vi "UserID.vi"(8 "Error In":errorcluster, 11 "Path In":path) -> (0 "Error Out":errorcluster, 1 "Student Info":T1, 3 "Path Out":path)   [LabVIEW 2014]
uses:
  Ctls/Student Info.ctl
  <vilib>/regexp/Match Regular Expression.xnode
panel:
  out "Subject Number":bool=TRUE
  out "Student Full Name":bool=TRUE
  out "Student Class Number":bool=TRUE
  out "Student ID":bool=TRUE
  out "Warning Text":string
  in  "Subject Number":string caption="Disciplina"
  in  "Student Class Number":string caption="Turma"
  in  "Student Full Name":string caption="Nome Completo"
  in  "Student ID":string caption="Número USP"
  in  "OK":bool
  # "Dados do Usuário"
  # "Verifique / Preencha os campos abaixo referentes aos dados do usuário:"
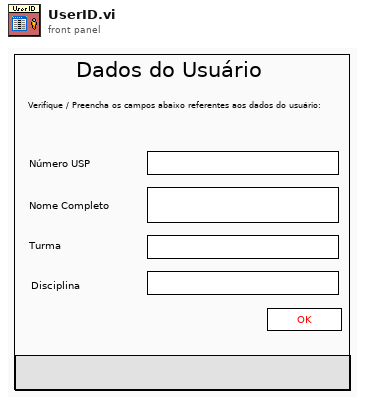
[diagram p1: front panel]
types:
  T1 = typedef "Student Info.ctl" = cluster{"Student ID":string, "Student Full Name":string, "Student Class Number":string, "Subject Number":string, "Last Online":string}
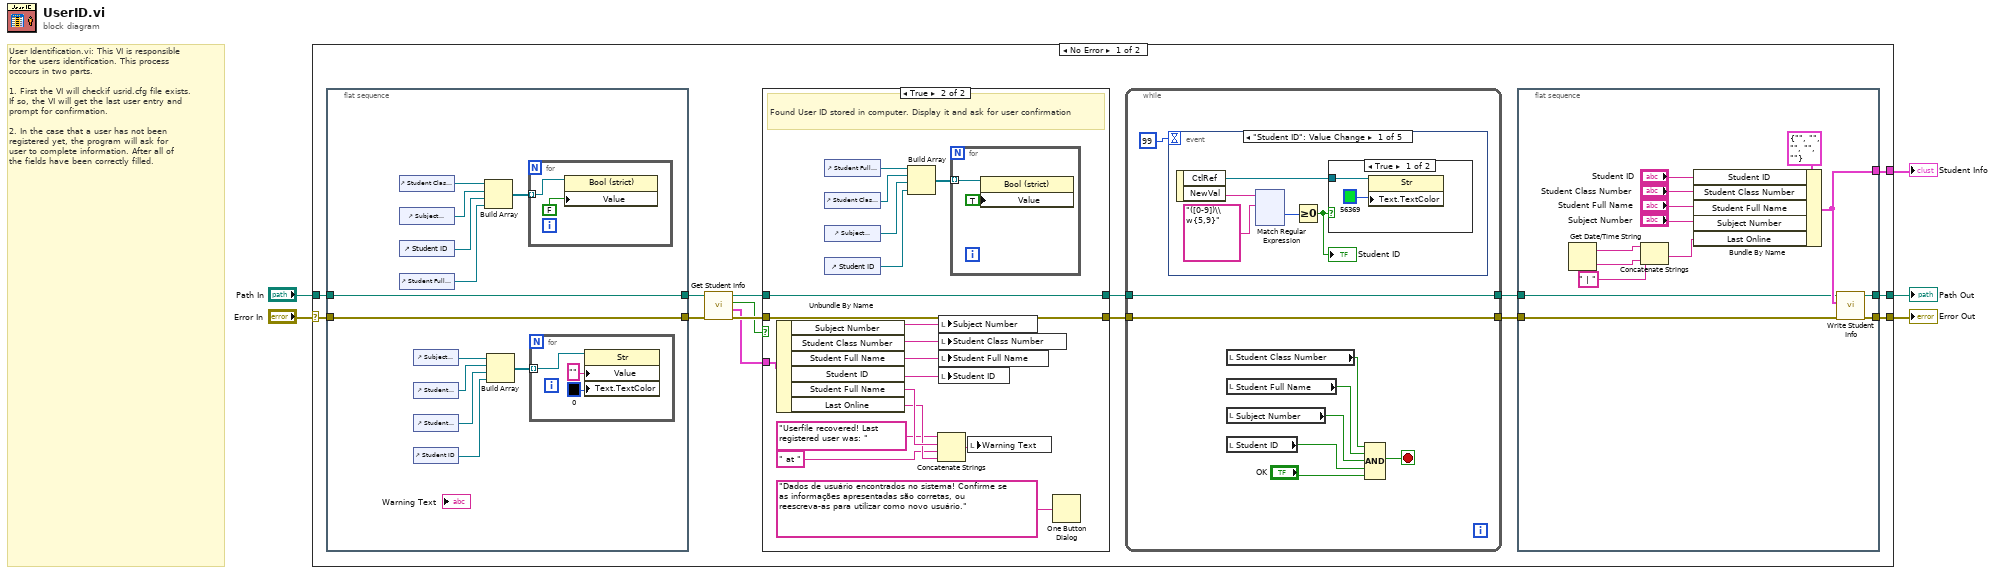
[diagram p0: block diagram]
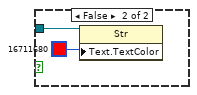
[diagram p2: hidden frame]
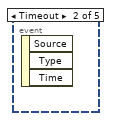
[diagram p3: hidden frame]
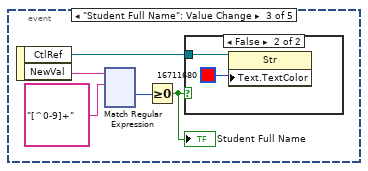
[diagram p4: hidden frame]
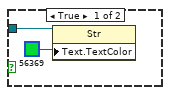
[diagram p5: hidden frame]
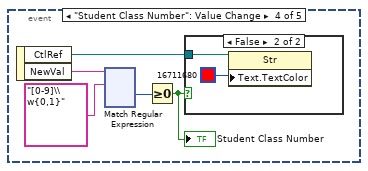
[diagram p6: hidden frame]
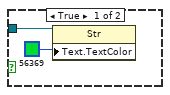
[diagram p7: hidden frame]
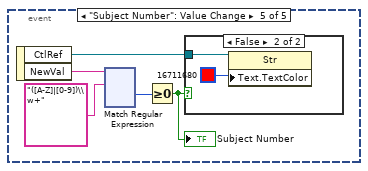
[diagram p8: hidden frame]
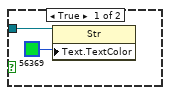
[diagram p9: hidden frame]
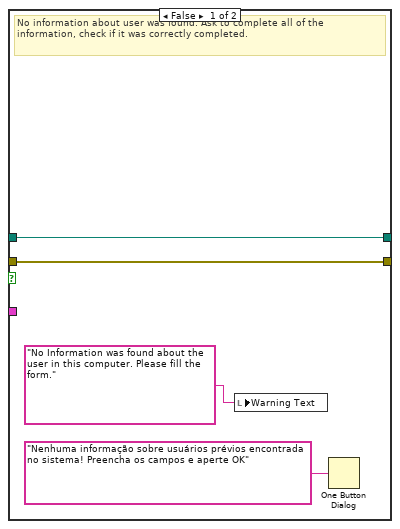
[diagram p10: hidden frame]
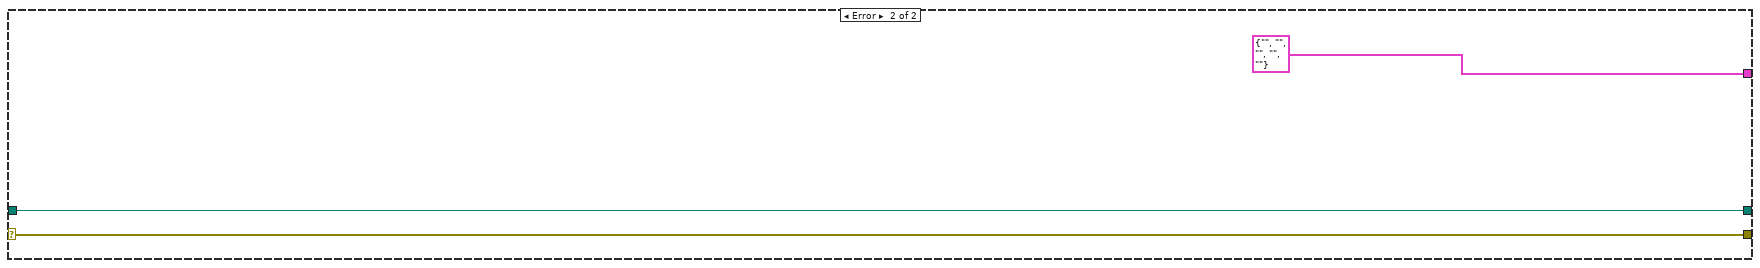
[diagram p11: hidden frame]
diagram:
  # "User Identification.vi: This VI is responsible \nfor the users identification. This process \noccours in two parts. \n\n1. First the VI will checkif usrid.cfg file exists.\nIf so, the VI will get the last user entry and \nprompt for confirmation.\n\n2. In the case that a user has not been \nregistered yet, the program will ask for\nuser to complete information. After all of \nthe fields have been correctly filled."
  n1 = case shown="No Error" "Error In" {
    selector: "Error In" -> [w15 w579]
    tunnel: [w11 w579] -> w5
    tunnel: "Path In" -> [w16 w578]
    tunnel: [w12 w578] -> w2
    tunnel: [w10 T1 {"Student ID"="", "Student Full Name"="", "Student Class Number"="", "Subject Number"="", "Last Online"=""} ("Student Info")] -> w1
    frame No Error {
      n2 = flat-sequence {
        tunnel: w16 -> [w537]
        tunnel: w15 -> [w536]
        tunnel: [w537] -> w14
        tunnel: [w536] -> w13
        frame #0 {
          n3 = control-ref of="Student Class Number"() -> (w541:refnum<vi>)
          n4 = control-ref of="Subject Number"() -> (w540:refnum<vi>)
          n5 = control-ref of="Student ID"() -> (w539:refnum<vi>)
          n6 = control-ref of="Student Full Name"() -> (w538:refnum<vi>)
          n7 = control-ref of="Subject Number"() -> (w545:refnum<vi>)
          n8 = control-ref of="Student Class Number"() -> (w544:refnum<vi>)
          n9 = control-ref of="Student Full Name"() -> (w543:refnum<vi>)
          n10 = control-ref of="Student ID"() -> (w542:refnum<vi>)
          n11 = Build Array(w541, w540, w539, w538) -> (w547:refnum<vi>[])
          n12 = Build Array(w545, w544, w543, w542) -> (w546:refnum<vi>[])
          n13 = for {
            tunnel: w547 -> [w549] mode=indexing
            n14 = property class="Bool (strict)"(reference=w549, "Value"=FALSE) -> ()  [unwired: 1 in, 2 out]
          }
          n15 = for {
            tunnel: w546 -> [w552] mode=indexing
            n16 = property class="Str"(reference=w552, "Value"="", "Text.TextColor"=u32 0) -> ()  [unwired: 1 in, 2 out]
          }
        }
      }
      n17 = call "Get Student Info.vi"("Error In"=w13, "Path In"=w14) -> ("Error Out"=w20:errorcluster, "Student Info"=w18:T1, "Found Usr Cfg File?"=w17:bool, "Path Out"=w19:path)  [unwired: 6 in]
      n18 = case shown="True" w17 {
        tunnel: [w555 w564] -> w9
        tunnel: w20 -> [w555 w564]
        tunnel: w19 -> [w556 w563]
        tunnel: w18 -> [_ w574]
        tunnel: [w556 w563] -> w8
        frame False {
          # "No information about user was found. Ask to complete all of the information, check if it was correctly completed."
          n19 = local write "Warning Text"("No Information was found about the user in this computer. Please fill the form." ("Warning Text")) -> ()
          n20 = One Button Dialog(message="Nenhuma informação sobre usuários prévios encontrada no sistema! Preencha os campos e aperte OK" ("regular expression")) -> ()  [unwired: 1 in, 1 out]
        }
        frame True {
          # "Found User ID stored in computer. Display it and ask for user confirmation"
          n21 = Unbundle By Name(w574) -> ("Subject Number"=w573:string, "Student Class Number"=w572:string, "Student Full Name"=w571:string, "Student ID"=w570:string, "Student Full Name"=w569:string, "Last Online"=w568:string)
          n22 = control-ref of="Student Full Name"() -> (w559:refnum<vi>)
          n23 = control-ref of="Student Class Number"() -> (w560:refnum<vi>)
          n24 = control-ref of="Subject Number"() -> (w561:refnum<vi>)
          n25 = control-ref of="Student ID"() -> (w562:refnum<vi>)
          n26 = Build Array(w559, w560, w561, w562) -> (w558:refnum<vi>[])
          n27 = Concatenate Strings("Userfile recovered! Last registered user was: ", w569, " at " ("string"), w568) -> (w565:string)
          n28 = local write "Subject Number"(w573) -> ()
          n29 = local write "Student Class Number"(w572) -> ()
          n30 = local write "Student Full Name"(w571) -> ()
          n31 = local write "Student ID"(w570) -> ()
          n32 = for {
            tunnel: w558 -> [w576] mode=indexing
            n33 = property class="Bool (strict)"(reference=w576, "Value"=TRUE) -> ()  [unwired: 1 in, 2 out]
          }
          n34 = local write "Warning Text"(w565) -> ()
          n35 = One Button Dialog(message="Dados de usuário encontrados no sistema! Confirme se as informações apresentadas são corretas, ou reescreva-as para utilizar como novo usuário." ("regular expression")) -> ()  [unwired: 1 in, 1 out]
        }
      }
      n36 = while {
        tunnel: w9 -> [w43]
        tunnel: [w43] -> w6
        tunnel: w8 -> [w40]
        tunnel: [w40] -> w7
        stop <- w41 stop-if-true
        n37 = event shown="[0] \"Student ID\": Value Change" {
          selector: _ -> [_ _ _ _ _]
          dyn-events: _ -> [_ _ _ _ _]
          timeout: 99 -> [_ _ _ _ _]
          event "Student ID": Value Change {
            n38 = event-data() -> ("CtlRef"=w48:refnum<vi>, "NewVal"=w44:string)  [unwired: 1 in]
            n39 = xnode "Match Regular Expression"("input string"=w44, "regular expression"="([0-9])\\w{5,9}") -> ("offset past match"=w45:i32)  [unwired: 4 in, 4 out]
            n40 = Greater Or Equal To 0?(x=w45) -> (x >= 0?=w46:bool)
            "Student ID" <- w46
            n41 = case shown="True" w46 {
              tunnel: w48 -> [w164 w165]
              frame True {
                n42 = property on="Property Node" class="Str"(reference=w164, "Text.TextColor"=u32 56369) -> ()  [unwired: 1 in, 2 out]
              }
              frame False {
                n43 = property on="Property Node" class="Str"(reference=w165, "Text.TextColor"=u32 16711680) -> ()  [unwired: 1 in, 2 out]
              }
            }
          }
          event Timeout {
            n44 = event-data() -> ()  [unwired: 1 in, 3 out]
          }
          event "Student Full Name": Value Change {
            n45 = event-data() -> ("CtlRef"=w168:refnum<vi>, "NewVal"=w169:string)  [unwired: 1 in]
            n46 = xnode "Match Regular Expression"("input string"=w169, "regular expression"="[^0-9]+") -> ("offset past match"=w170:i32)  [unwired: 4 in, 4 out]
            n47 = Greater Or Equal To 0?(x=w170) -> (x >= 0?=w167:bool)
            "Student Full Name" <- w167
            n48 = case shown="False" w167 {
              tunnel: w168 -> [w173 w174]
              frame True {
                n49 = property on="Property Node" class="Str"(reference=w173, "Text.TextColor"=u32 56369) -> ()  [unwired: 1 in, 2 out]
              }
              frame False {
                n50 = property on="Property Node" class="Str"(reference=w174, "Text.TextColor"=u32 16711680) -> ()  [unwired: 1 in, 2 out]
              }
            }
          }
          event "Student Class Number": Value Change {
            n51 = event-data() -> ("CtlRef"=w291:refnum<vi>, "NewVal"=w293:string)  [unwired: 1 in]
            n52 = xnode "Match Regular Expression"("input string"=w293, "regular expression"="[0-9]\\w{0,1}") -> ("offset past match"=w292:i32)  [unwired: 4 in, 4 out]
            n53 = Greater Or Equal To 0?(x=w292) -> (x >= 0?=w290:bool)
            "Student Class Number" <- w290
            n54 = case shown="False" w290 {
              tunnel: w291 -> [w296 w297]
              frame True {
                n55 = property on="Property Node" class="Str"(reference=w296, "Text.TextColor"=u32 56369) -> ()  [unwired: 1 in, 2 out]
              }
              frame False {
                n56 = property on="Property Node" class="Str"(reference=w297, "Text.TextColor"=u32 16711680) -> ()  [unwired: 1 in, 2 out]
              }
            }
          }
          event "Subject Number": Value Change {
            n57 = event-data() -> ("CtlRef"=w414:refnum<vi>, "NewVal"=w416:string)  [unwired: 1 in]
            n58 = xnode "Match Regular Expression"("input string"=w416, "regular expression"="([A-Z]|[0-9])\\w+") -> ("offset past match"=w415:i32)  [unwired: 4 in, 4 out]
            n59 = Greater Or Equal To 0?(x=w415) -> (x >= 0?=w413:bool)
            "Subject Number" <- w413
            n60 = case shown="False" w413 {
              tunnel: w414 -> [w419 w420]
              frame True {
                n61 = property on="Property Node" class="Str"(reference=w419, "Text.TextColor"=u32 56369) -> ()  [unwired: 1 in, 2 out]
              }
              frame False {
                n62 = property on="Property Node" class="Str"(reference=w420, "Text.TextColor"=u32 16711680) -> ()  [unwired: 1 in, 2 out]
              }
            }
          }
        }
        n63 = local read "Student Class Number"() -> (w36:bool)
        n64 = local read "Student Full Name"() -> (w37:bool)
        n65 = local read "Subject Number"() -> (w38:bool)
        n66 = local read "Student ID"() -> (w39:bool)
        n67 = Compound Arithmetic op=AND(w36, w37, w38, w39, "OK") -> (w41:bool)
      }
      n68 = flat-sequence {
        tunnel: [w25] -> w12
        tunnel: [w24] -> w11
        tunnel: [w23] -> w10
        tunnel: w7 -> [w22]
        tunnel: w6 -> [w21]
        frame #0 {
          n69 = Get Date/Time String() -> (date string=w29:string, time string=w28:string)  [unwired: 3 in]
          n70 = Concatenate Strings(w29, " | " ("string"), w28) -> (w27:string)
          n71 = Bundle By Name(cluster=T1 {"Student ID"="", "Student Full Name"="", "Student Class Number"="", "Subject Number"="", "Last Online"=""} ("Student Info"), "Student ID"="Student ID", "Student Class Number"="Student Class Number", "Student Full Name"="Student Full Name", "Subject Number"="Subject Number", "Last Online"=w27) -> (w23:T1)
          n72 = call "Write Student Info.vi"("Error In"=w21, "Student Info"=w23, "Path In"=w22) -> ("Error Out"=w24:errorcluster, "Path Out"=w25:path)  [unwired: 7 in]
        }
      }
    }
    frame Error {
    }
  }
  "Error Out" <- w5
  "Path Out" <- w2
  "Student Info" <- w1
